vi "Mode Reference.vi"(0 "Sample Test Template in":refnum<class "Sample Test Template.lvclass">, 11 "Error in":errorcluster) -> (4 "Sample Test Template out":refnum<class "Sample Test Template.lvclass">, 6 "VI Refnum":refnum<vi>, 15 "Error out":errorcluster)   [LabVIEW 2020, in "Sample Test Template.lvclass"]
doc: "Dynamic method for mode page reference"
uses:
  Sample Test Template.lvclass
  Parent/Typedef/LV2 Control.ctl
  Mode Page.vi
  Parent/Test.lvclass
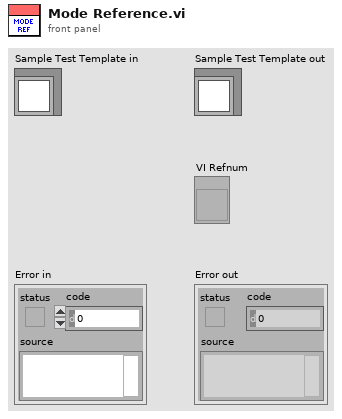
[diagram p1: front panel]
types:
  T1 = typedef "Test.lvclass/LV2 Control.ctl" = enum16{"Home", "Mode", "Config", "Status", "Read"}
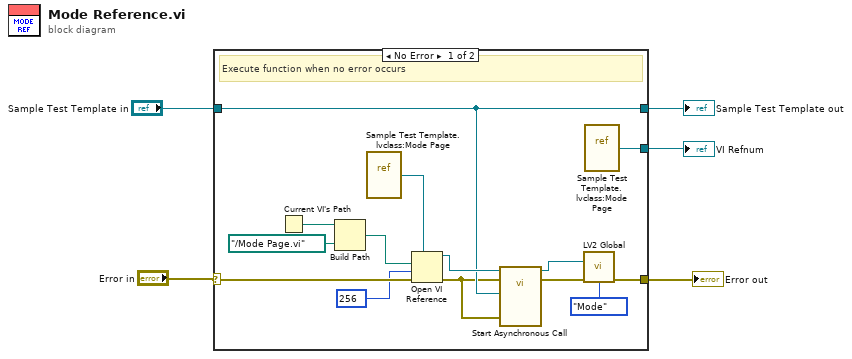
[diagram p0: block diagram]
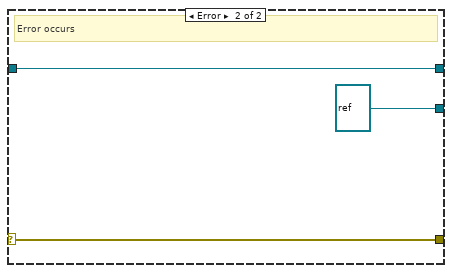
[diagram p2: hidden frame]
diagram:
  n1 = case shown="No Error" "Error in" {
    selector: "Error in" -> [w19 w22]
    tunnel: [w7 w22] -> w3
    tunnel: [w18 refnum<vi> refnum] -> w1
    tunnel: "Sample Test Template in" -> [w11 w20]
    tunnel: [w11 w20] -> w2
    frame No Error {
      # "Execute function when no error occurs"
      n2 = Current VI's Path() -> (path=w17:path)
      n3 = Build Path(base path=w17, name or relative path=path "../Mode Page.vi") -> (appended path=w15:path)
      n4 = vi-ref "Sample Test Template.lvclass:Mode Page.vi"() -> (w14:refnum<vi>)
      n5 = Open VI Reference(type specifier VI Refnum (for type only)=w14, vi path=w15, options=256, error in (no error)=w19) -> (vi reference=w12:refnum<vi>, error out=w10:errorcluster)  [unwired: 2 in]
      n6 = call-by-ref "Start Asynchronous Call"(reference=w12, error in=w10, "Error In"=w10, "Sample Test Template in"=w11) -> (reference out=w6:refnum<vi>, error out=w9:errorcluster)  [unwired: 8 in, 2 out]
      n7 = call "LV2 Global.vi"("Mode Ref In"=w6, "Error In"=w9, "Enum"=LV2_Control."Mode") -> ("Error Out"=w7:errorcluster)  [unwired: 8 in, 4 out]
      n8 = vi-ref "Sample Test Template.lvclass:Mode Page.vi"() -> (w18:refnum<vi>)
    }
    frame Error {
      # "Error occurs"
    }
  }
  "Error out" <- w3
  "Sample Test Template out" <- w2
  "VI Refnum" <- w1
